vi "phase array(antena).vi"() -> ()   [LabVIEW 2017]
panel:
  out "Beam width":dbl
  out "phi(degree)":dbl
  in  "Delay phase(degree)":dbl
  in  "Error Rate % (d)":dbl
  in  "Number of element":dbl
  out "Polar Plot":picture caption="Ploar Plot"
  in  "Plot Color":u32(colorbox)=16715776
  in  "Grid Color":u32(colorbox)
  in  "Visible Section":u16(ring)=8
  # "Phase array Options"
  # "Cosmetic Options"
  # "Data result"
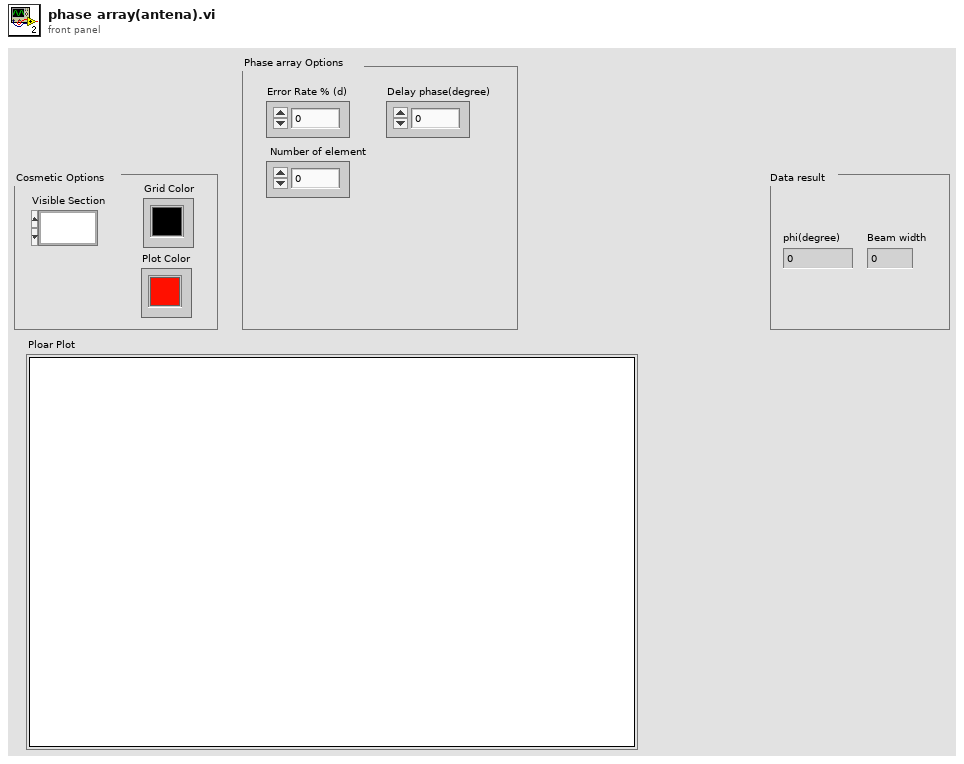
[diagram p1: front panel]
types:
  T1 = cluster{"maximum":dbl, "minimum":dbl, "clip to min":bool, "log?(F)":bool, "grid color":u32, "plot color":u32, "format and precision":cluster{"format":enum8{"Decimal", "Scientific", "Engineering", "Binary", "Octal", "Hex"}, "precision":u8}, "visible section":u16}
  T2 = typedef "LVBoundsTypeDef.ctl" = cluster{"Width":u32, "Height":u32}
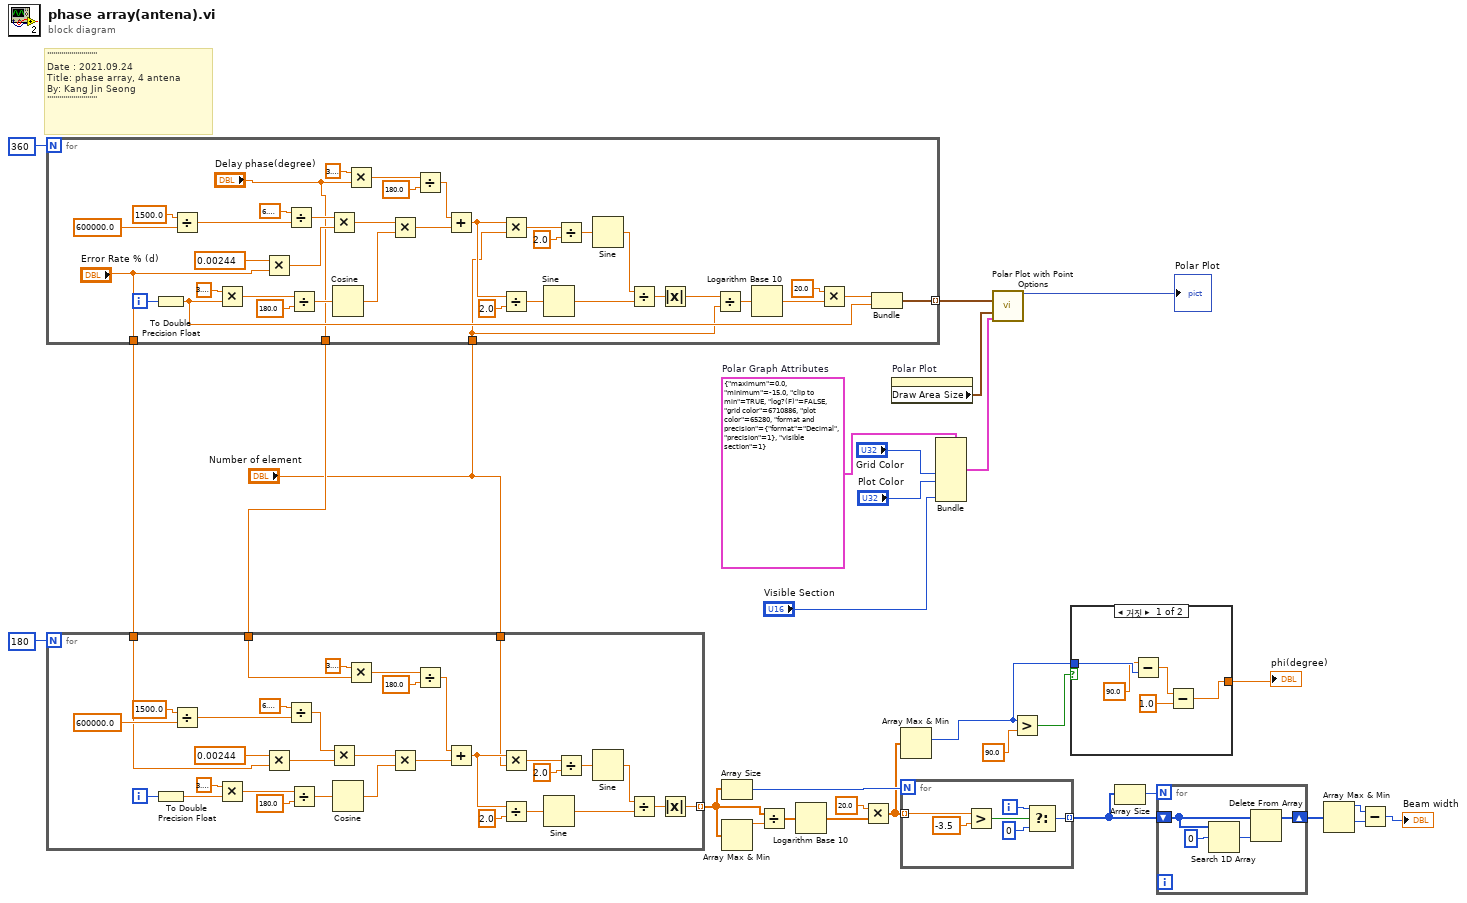
[diagram p0: block diagram]
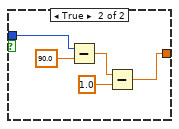
[diagram p2: hidden frame]
diagram:
  w30 = T1 {"maximum"=0.0, "minimum"=-15.0, "clip to min"=TRUE, "log?(F)"=FALSE, "grid color"=6710886, "plot color"=65280, "format and precision"={"format"=enum."Decimal", "precision"=1}, "visible section"=1}  # Polar Graph Attributes
  # "'''''''''''''''''''''''''\nDate : 2021.09.24\nTitle: phase array, 4 antena\nBy: Kang Jin Seong\n'''''''''''''''''''''''''"
  n1 = for {
    N: 360 -> [_]
    tunnel: [w62] -> w23 mode=indexing
    tunnel: ["Delay phase(degree)"] -> w8
    tunnel: ["Error Rate % (d)"] -> w7
    tunnel: "Number of element" -> [w33]
    i -> [w34]
    n2 = To Double Precision Float(number=w34) -> (double precision float=w36:dbl)
    n3 = Divide(x=1500.0, y=600000.0) -> (x/y=w57:dbl)
    n4 = Multiply(x=3.141592653589793, y=w36) -> (x*y=w67:dbl)
    n5 = Multiply(x=0.00244 ("y"), y="Error Rate % (d)") -> (x*y=w54:dbl)
    n6 = Divide(x=6.283185307179586, y=w57) -> (x/y=w56:dbl)
    n7 = Divide(x=w67, y=180.0) -> (x/y=w65:dbl)
    n8 = Multiply(x=w56, y=w54) -> (x*y=w64:dbl)
    n9 = Cosine(x=w65) -> (cos(x)=w61:dbl)
    n10 = Multiply(x=3.141592653589793, y="Delay phase(degree)") -> (x*y=w44:dbl)
    n11 = Multiply(x=w64, y=w61) -> (x*y=w46:dbl)
    n12 = Divide(x=w44, y=180.0) -> (x/y=w42:dbl)
    n13 = Add(x=w42, y=w46) -> (x+y=w51:dbl)
    n14 = Multiply(x=w51, y=w33) -> (x*y=w53:dbl)
    n15 = Divide(x=w51, y=2.0) -> (x/y=w49:dbl)
    n16 = Sine(x=w49) -> (sin(x)=w47:dbl)
    n17 = Divide(x=w53, y=2.0) -> (x/y=w52:dbl)
    n18 = Sine(x=w52) -> (sin(x)=w48:dbl)
    n19 = Divide(x=w48, y=w47) -> (x/y=w38:dbl)
    n20 = Absolute Value(x=w38) -> (abs(x)=w37:dbl)
    n21 = Divide(x=w37, y=w33) -> (x/y=w41:dbl)
    n22 = Logarithm Base 10(1:w41) -> (0:w40:dbl)
    n23 = Multiply(x=20.0, y=w40) -> (x*y=w35:dbl)
    n24 = Bundle(w35, w36) -> (w62:cluster{dbl, dbl})  [unwired: 1 in]
  }
  n25 = for {
    N: 180 -> [_]
    tunnel: [w72] -> w13 mode=indexing
    tunnel: w8 -> [w71]
    tunnel: w7 -> [w70]
    tunnel: "Number of element" -> [w69]
    i -> [w73]
    n26 = To Double Precision Float(number=w73) -> (double precision float=w74:dbl)
    n27 = Divide(x=1500.0, y=600000.0) -> (x/y=w91:dbl)
    n28 = Multiply(x=3.141592653589793, y=w74) -> (x*y=w100:dbl)
    n29 = Multiply(x=0.00244 ("y"), y=w70) -> (x*y=w88:dbl)
    n30 = Divide(x=6.283185307179586, y=w91) -> (x/y=w90:dbl)
    n31 = Divide(x=w100, y=180.0) -> (x/y=w98:dbl)
    n32 = Multiply(x=w90, y=w88) -> (x*y=w97:dbl)
    n33 = Cosine(x=w98) -> (cos(x)=w95:dbl)
    n34 = Multiply(x=3.141592653589793, y=w71) -> (x*y=w78:dbl)
    n35 = Multiply(x=w97, y=w95) -> (x*y=w80:dbl)
    n36 = Divide(x=w78, y=180.0) -> (x/y=w76:dbl)
    n37 = Add(x=w76, y=w80) -> (x+y=w85:dbl)
    n38 = Multiply(x=w85, y=w69) -> (x*y=w87:dbl)
    n39 = Divide(x=w85, y=2.0) -> (x/y=w83:dbl)
    n40 = Sine(x=w83) -> (sin(x)=w81:dbl)
    n41 = Divide(x=w87, y=2.0) -> (x/y=w86:dbl)
    n42 = Sine(x=w86) -> (sin(x)=w82:dbl)
    n43 = Divide(x=w82, y=w81) -> (x/y=w75:dbl)
    n44 = Absolute Value(x=w75) -> (abs(x)=w72:dbl)
  }
  n45 = Array Size(array=w13) -> (size(s)=w12:i32)
  n46 = Array Max & Min(array=w13) -> (max value=w17:dbl)  [unwired: 3 out]
  n47 = Divide(x=w13, y=w17) -> (x/y=w16:dbl[])
  n48 = Logarithm Base 10(1:w16) -> (0:w15:dbl[])
  n49 = Multiply(x=20.0, y=w15) -> (x*y=w9:dbl[])
  n50 = property on="Polar Plot" class="Pict"() -> ("Draw Area Size"=w24:T2)  [unwired: 2 in, 2 out]
  n51 = Array Max & Min(array=w9) -> (max index (indices)=w4:i32)  [unwired: 3 out]
  n52 = for {
    N: w12 -> [_]
    tunnel: w9 -> [w104] mode=indexing
    tunnel: [w103] -> w11 mode=indexing
    i -> [w102]
    n53 = Greater?(x=w104, y=-3.5) -> (0:w106:bool)
    n54 = Select(t=w102, s=w106, f=0) -> (s? t:f=w103:i32)
  }
  n55 = Bundle(cluster=w30, "grid color"="Grid Color", "plot color"="Plot Color", "visible section"="Visible Section") -> (w29:T1)  [unwired: 5 in]
  n56 = call <vilib>:"Polar Plot with Point Options.vi"("data array [mag, phase (deg)]"=w23, "dimensions (w,h)"=w24, "polar attributes"=w29) -> ("new picture"=→"Polar Plot":picture)  [unwired: 12 in]
  n57 = Greater?(x=w4, y=90.0) -> (0:w5:bool)
  n58 = case shown="거짓" w5 {
    tunnel: w4 -> [w112 w117]
    tunnel: [w108 w113] -> w1
    frame False {
      n59 = Subtract(x=90.0, y=w112) -> (x-y=w110:dbl)
      n60 = Subtract(x=w110, y=1.0) -> (x-y=w108:dbl)
    }
    frame True {
      n61 = Subtract(x=w117, y=90.0) -> (x-y=w115:dbl)
      n62 = Subtract(x=w115, y=1.0) -> (x-y=w113:dbl)
    }
  }
  "phi(degree)" <- w1
  n63 = Array Size(array=w11) -> (size(s)=w20:i32)
  n64 = for {
    N: w20 -> [_]
    shift-right: [w120] -> w10
    shift-left: w11 -> [w119]
    n65 = Search 1D Array(1D array=w119, element=0 ("원소")) -> (index of element=w121:i32)  [unwired: 1 in]
    n66 = Delete From Array(array=w119, index=w121) -> (array with subset deleted=w120:i32[])  [unwired: 1 in, 1 out]
  }
  n67 = Array Max & Min(array=w10) -> (max value=w19:i32, min value=w18:i32)  [unwired: 2 out]
  n68 = Subtract(x=w19, y=w18) -> (x-y=→"Beam width":i32)
